vi "ControlShooter.vi"(1 "State":T2) -> (0 "To Shooter\nSolenoid Loop":T1=enum."Forward")   [LabVIEW 2013]
uses:
  typedefs/subStates.ctl
  <vilib>/Rock Robotics/WPI/Solenoid/WPI_SolenoidValue.ctl
  typedefs/fg_typedef.ctl
  <vilib>/Rock Robotics/WPI/Solenoid/WPI_SolenoidGetEnum.vi
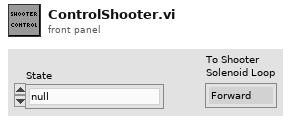
[diagram p1: front panel]
types:
  T1 = typedef "WPI_SolenoidValue.ctl" = enum16{"Off", "On", "Forward", "Reverse"}
  T2 = typedef "subStates.ctl" = enum16{"null", "wait", "driver control", "auto", "manual override", "hold position", "rotate", "pickup", "pass", "load", "goto shoot", "shoot", "end"}
  T3 = typedef "fg_typedef.ctl" = enum16{"Get", "Set"}
  T4 = typedef "WPI_DigitalInputDevRef.ctl" = cluster{"DevStatus":errorcluster, "DIO Channel":T5, "Digital Module":T6}
  T5 = typedef "FPGA_DIOChannel.ctl" = enum8{"DIO 1", "DIO 2", "DIO 3", "DIO 4", "DIO 5", "DIO 6", "DIO 7", "DIO 8", "DIO 9", "DIO 10", "DIO 11", "DIO 12", "DIO 13", "DIO 14", "Invalid"}
  T6 = typedef "FPGA_TypedefDigitalModule.ctl" = enum16{"Digital Module 1", "Digital Module 2"}
  T7 = typedef "WPI_SolenoidDevRef.ctl" = cluster{"DevStatus":errorcluster, "Solenoid Module":T8, "Forward Solenoid Channel":T9, "Reverse Solenoid Channel":T9}
  T8 = typedef "FPGA_TypedefSolenoidModule.ctl" = enum16{"Solenoid Module 1", "Solenoid Module 2"}
  T9 = typedef "WPI_SolenoidChannel.ctl" = enum8{"Solenoid 1", "Solenoid 2", "Solenoid 3", "Solenoid 4", "Solenoid 5", "Solenoid 6", "Solenoid 7", "Solenoid 8", "Invalid"}
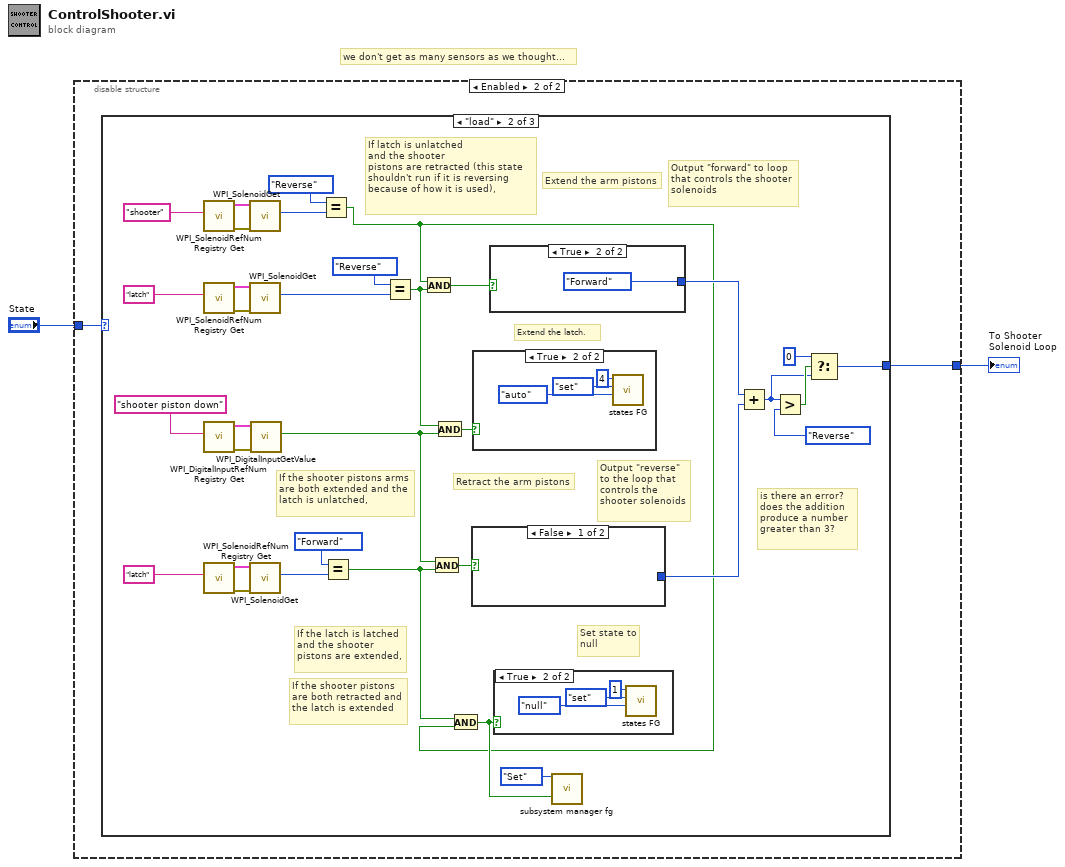
[diagram p0: block diagram]
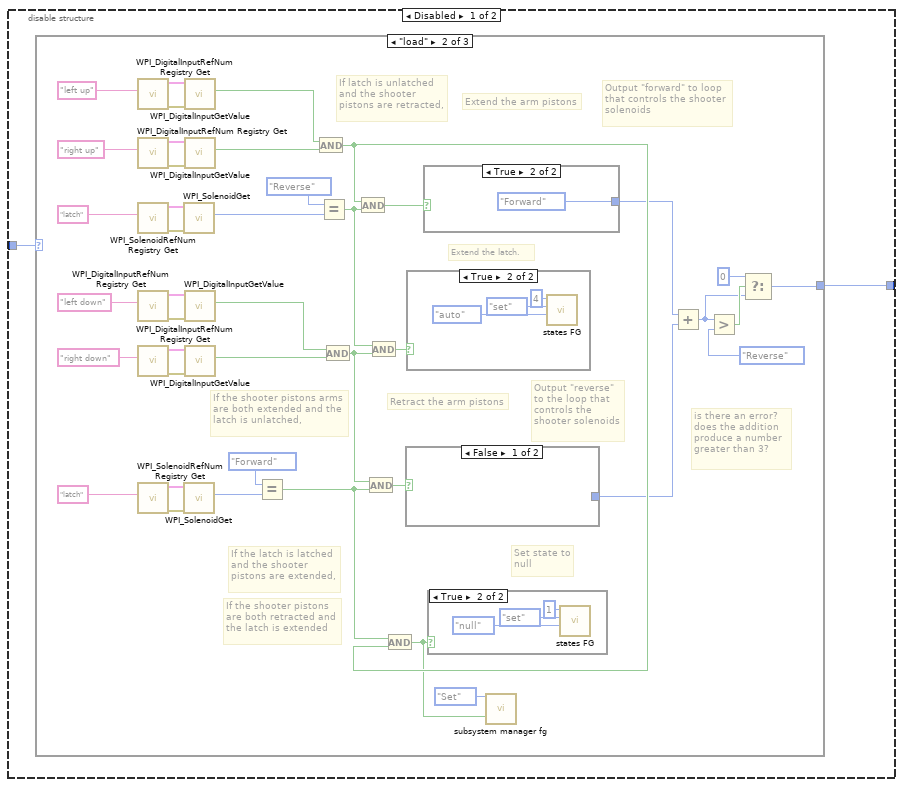
[diagram p2: hidden frame]
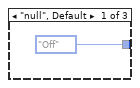
[diagram p3: hidden frame]
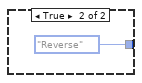
[diagram p5: hidden frame]
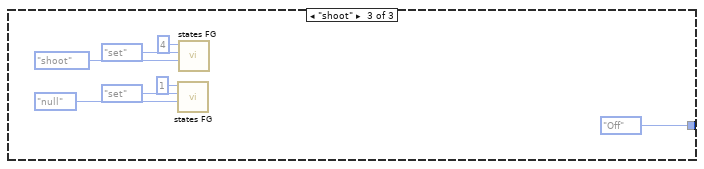
[diagram p8: hidden frame]
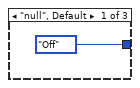
[diagram p9: hidden frame]
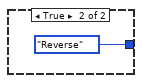
[diagram p11: hidden frame]
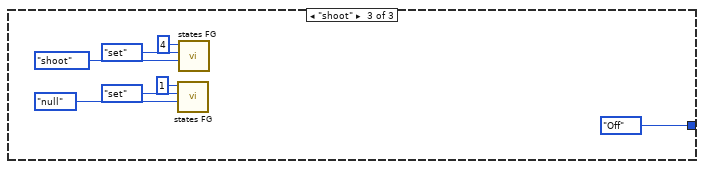
[diagram p14: hidden frame]
diagram:
  # "we don't get as many sensors as we thought..."
  n1 = disable-structure shown="Enabled" {
    disable-tunnel: "State" -> [w4 w64]
    disable-tunnel: [w3 w63] -> w1
    frame Disabled {
      n2 = case shown="\"load\"" w4 {
        tunnel: [WPI_SolenoidValue."Off" ("To Shooter\nSolenoid Loop") w9 WPI_SolenoidValue."Off" ("To Shooter\nSolenoid Loop")] -> w3
        frame "null", Default {
        }
        frame "load" {
          # "is there an error?\ndoes the addition\nproduce a number \ngreater than 3?"
          # "Output \"reverse\"\nto the loop that\ncontrols the\nshooter solenoids"
          # "Output \"forward\" to loop\nthat controls the shooter\nsolenoids"
          # "Set state to\nnull"
          # "If the shooter pistons\nare both retracted and\nthe latch is extended"
          # "If the latch is latched\nand the shooter\npistons are extended,"
          # "Retract the arm pistons"
          # "If latch is unlatched\nand the shooter\npistons are retracted,"
          # "Extend the latch."
          # "If the shooter pistons arms\nare both extended and the\nlatch is unlatched,"
          # "Extend the arm pistons"
          n3 = call <vilib>:"WPI_DigitalInputRefNum Registry Get.vi"("refnum name"="left up") -> ("error out"=w38:errorcluster, "DigitalInputDevRef"=w39:T4)  [unwired: 9 in]
          n4 = call <vilib>:"WPI_DigitalInputRefNum Registry Get.vi"("refnum name"="right up") -> ("error out"=w41:errorcluster, "DigitalInputDevRef"=w42:T4)  [unwired: 9 in]
          n5 = call <vilib>:"WPI_SolenoidRefNum Registry Get.vi"("refnum name"="latch") -> ("error out"=w47:errorcluster, "SolenoidDevRef"=w46:T7)  [unwired: 9 in]
          n6 = call <vilib>:"WPI_DigitalInputRefNum Registry Get.vi"("refnum name"="left down") -> ("error out"=w31:errorcluster, "DigitalInputDevRef"=w32:T4)  [unwired: 9 in]
          n7 = call <vilib>:"WPI_DigitalInputRefNum Registry Get.vi"("refnum name"="right down") -> ("error out"=w28:errorcluster, "DigitalInputDevRef"=w29:T4)  [unwired: 9 in]
          n8 = call <vilib>:"WPI_SolenoidRefNum Registry Get.vi"("refnum name"="latch") -> ("error out"=w24:errorcluster, "SolenoidDevRef"=w23:T7)  [unwired: 9 in]
          n9 = call-poly <vilib>:"WPI_SolenoidGet.vi"("error in (no error)"=w47, "SolenoidDevRef"=w46) -> ("Value"=w44:T1)  [unwired: 7 in, 2 out]
          n10 = call-poly <vilib>:"WPI_SolenoidGet.vi"("error in (no error)"=w24, "SolenoidDevRef"=w23) -> ("Value"=w21:T1)  [unwired: 7 in, 2 out]
          n11 = call <vilib>:"WPI_DigitalInputGetValue.vi"("error in (no error)"=w38, "DigitalInputDevRef"=w39) -> ("Value"=w36:bool)  [unwired: 7 in, 2 out]
          n12 = call <vilib>:"WPI_DigitalInputGetValue.vi"("error in (no error)"=w41, "DigitalInputDevRef"=w42) -> ("Value"=w35:bool)  [unwired: 7 in, 2 out]
          n13 = call <vilib>:"WPI_DigitalInputGetValue.vi"("error in (no error)"=w31, "DigitalInputDevRef"=w32) -> ("Value"=w26:bool)  [unwired: 7 in, 2 out]
          n14 = call <vilib>:"WPI_DigitalInputGetValue.vi"("error in (no error)"=w28, "DigitalInputDevRef"=w29) -> ("Value"=w25:bool)  [unwired: 7 in, 2 out]
          n15 = Equal?(x=WPI_SolenoidValue."Forward", y=w21) -> (x = y?=w16:bool)
          n16 = And(x=w36, y=w35) -> (x .and. y?=w15:bool)
          n17 = Equal?(x=WPI_SolenoidValue."Reverse", y=w44) -> (x = y?=w17:bool)
          n18 = And(x=w26, y=w25) -> (x .and. y?=w18:bool)
          n19 = And(x=w15, y=w17) -> (x .and. y?=w34:bool)
          n20 = And(x=w18, y=w16) -> (x .and. y?=w19:bool)
          n21 = And(x=w17, y=w18) -> (x .and. y?=w33:bool)
          n22 = And(x=w16, y=w15) -> (x .and. y?=w6:bool)
          n23 = case shown="False" w19 {
            tunnel: [_ WPI_SolenoidValue."Reverse" ("Value")] -> w8
            frame False {
            }
            frame True {
            }
          }
          n24 = case shown="True" w33 {
            frame False {
            }
            frame True {
              n25 = call "states FG.vi"("subState in"=subStates."auto", "menu (get)"=enum16{"set", "get"}."set", "Loop ID"=4) -> ()  [unwired: 5 in, 4 out]
            }
          }
          n26 = case shown="True" w34 {
            tunnel: [_ WPI_SolenoidValue."Forward" ("Value")] -> w14
            frame False {
            }
            frame True {
            }
          }
          n27 = case shown="True" w6 {
            frame False {
            }
            frame True {
              n28 = call "states FG.vi"("subState in"=subStates."null", "menu (get)"=enum16{"set", "get"}."set", "Loop ID"=1) -> ()  [unwired: 5 in, 4 out]
            }
          }
          n29 = call "subsystem manager fg.vi"("Menu"=fg_typedef."Set", "Shooter Cocked"=w6) -> ()  [unwired: 13 in, 5 out]
          n30 = Add(x=w14, y=w8) -> (x+y=w11:u16)
          n31 = Greater?(x=w11, y=WPI_SolenoidValue."Reverse" ("Value")) -> (0:w12:bool)
          n32 = Select(t=0, s=w12, f=w11) -> (s? t:f=w9:i32)
        }
        frame "shoot" {
          n33 = call "states FG.vi"("subState in"=subStates."null", "menu (get)"=enum16{"set", "get"}."set", "Loop ID"=1) -> ()  [unwired: 5 in, 4 out]
          n34 = call "states FG.vi"("subState in"=subStates."shoot", "menu (get)"=enum16{"set", "get"}."set", "Loop ID"=4) -> ()  [unwired: 5 in, 4 out]
        }
      }
    }
    frame Enabled {
      n35 = case shown="\"load\"" w64 {
        tunnel: [WPI_SolenoidValue."Off" ("To Shooter\nSolenoid Loop") w76 WPI_SolenoidValue."Off" ("To Shooter\nSolenoid Loop")] -> w63
        frame "null", Default {
        }
        frame "load" {
          # "is there an error?\ndoes the addition\nproduce a number \ngreater than 3?"
          # "Output \"reverse\"\nto the loop that\ncontrols the\nshooter solenoids"
          # "Output \"forward\" to loop\nthat controls the shooter\nsolenoids"
          # "Set state to\nnull"
          # "If the shooter pistons\nare both retracted and\nthe latch is extended"
          # "If the latch is latched\nand the shooter\npistons are extended,"
          # "Retract the arm pistons"
          # "If latch is unlatched\nand the shooter\npistons are retracted (this state shouldn't run if it is reversing because of how it is used),"
          # "Extend the latch."
          # "If the shooter pistons arms\nare both extended and the\nlatch is unlatched,"
          # "Extend the arm pistons"
          n36 = call <vilib>:"WPI_SolenoidRefNum Registry Get.vi"("refnum name"="shooter") -> ("error out"=w68:errorcluster, "SolenoidDevRef"=w69:T7)  [unwired: 9 in]
          n37 = call <vilib>:"WPI_SolenoidRefNum Registry Get.vi"("refnum name"="latch") -> ("error out"=w99:errorcluster, "SolenoidDevRef"=w98:T7)  [unwired: 9 in]
          n38 = call <vilib>:"WPI_DigitalInputRefNum Registry Get.vi"("refnum name"="shooter piston down") -> ("error out"=w91:errorcluster, "DigitalInputDevRef"=w92:T4)  [unwired: 9 in]
          n39 = call <vilib>:"WPI_SolenoidRefNum Registry Get.vi"("refnum name"="latch") -> ("error out"=w89:errorcluster, "SolenoidDevRef"=w88:T7)  [unwired: 9 in]
          n40 = call-poly <vilib>:"WPI_SolenoidGet.vi"("error in (no error)"=w68, "SolenoidDevRef"=w69) -> ("Value"=w70:T1)  [unwired: 7 in, 2 out]
          n41 = call-poly <vilib>:"WPI_SolenoidGet.vi"("error in (no error)"=w99, "SolenoidDevRef"=w98) -> ("Value"=w96:T1)  [unwired: 7 in, 2 out]
          n42 = call-poly <vilib>:"WPI_SolenoidGet.vi"("error in (no error)"=w89, "SolenoidDevRef"=w88) -> ("Value"=w86:T1)  [unwired: 7 in, 2 out]
          n43 = call <vilib>:"WPI_DigitalInputGetValue.vi"("error in (no error)"=w91, "DigitalInputDevRef"=w92) -> ("Value"=w72:bool)  [unwired: 7 in, 2 out]
          n44 = Equal?(x=WPI_SolenoidValue."Reverse", y=w70) -> (x = y?=w66:bool)
          n45 = Equal?(x=WPI_SolenoidValue."Forward", y=w86) -> (x = y?=w82:bool)
          n46 = Equal?(x=WPI_SolenoidValue."Reverse", y=w96) -> (x = y?=w83:bool)
          n47 = And(x=w66, y=w83) -> (x .and. y?=w94:bool)
          n48 = And(x=w72, y=w82) -> (x .and. y?=w84:bool)
          n49 = And(x=w83, y=w72) -> (x .and. y?=w93:bool)
          n50 = And(x=w82, y=w66) -> (x .and. y?=w73:bool)
          n51 = case shown="False" w84 {
            tunnel: [_ WPI_SolenoidValue."Reverse" ("Value")] -> w75
            frame False {
            }
            frame True {
            }
          }
          n52 = case shown="True" w93 {
            frame False {
            }
            frame True {
              n53 = call "states FG.vi"("subState in"=subStates."auto", "menu (get)"=enum16{"set", "get"}."set", "Loop ID"=4) -> ()  [unwired: 5 in, 4 out]
            }
          }
          n54 = case shown="True" w94 {
            tunnel: [_ WPI_SolenoidValue."Forward" ("Value")] -> w81
            frame False {
            }
            frame True {
            }
          }
          n55 = case shown="True" w73 {
            frame False {
            }
            frame True {
              n56 = call "states FG.vi"("subState in"=subStates."null", "menu (get)"=enum16{"set", "get"}."set", "Loop ID"=1) -> ()  [unwired: 5 in, 4 out]
            }
          }
          n57 = call "subsystem manager fg.vi"("Menu"=fg_typedef."Set", "Shooter Cocked"=w73) -> ()  [unwired: 13 in, 5 out]
          n58 = Add(x=w81, y=w75) -> (x+y=w78:u16)
          n59 = Greater?(x=w78, y=WPI_SolenoidValue."Reverse" ("Value")) -> (0:w79:bool)
          n60 = Select(t=0, s=w79, f=w78) -> (s? t:f=w76:i32)
        }
        frame "shoot" {
          n61 = call "states FG.vi"("subState in"=subStates."null", "menu (get)"=enum16{"set", "get"}."set", "Loop ID"=1) -> ()  [unwired: 5 in, 4 out]
          n62 = call "states FG.vi"("subState in"=subStates."shoot", "menu (get)"=enum16{"set", "get"}."set", "Loop ID"=4) -> ()  [unwired: 5 in, 4 out]
        }
      }
    }
  }
  "To Shooter\nSolenoid Loop" <- w1
